vi "Tree_insert tag.vi"(0 "ChannelTree":refnum<vi>, 5 "Active Item:Tag":string, 7 "Left Cell String":string, 9 "Child Text":string[](array[string]), 11 "error in (no error)":errorcluster, 12 "Child Tag":string, 13 "Indent Level (-1 same as ActiveTag)":i32=-1) -> (4 "dup ChannelTree":refnum<vi>, 6 "Active Item:Tag out":string, 8 "Child Position":i32, 15 "error out":errorcluster)   [LabVIEW 2014]
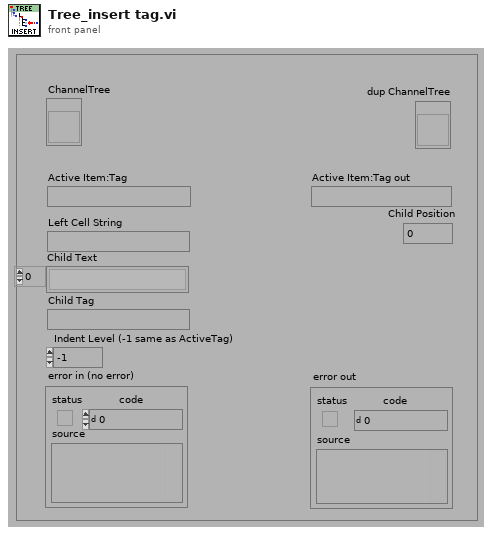
[diagram p1: front panel]
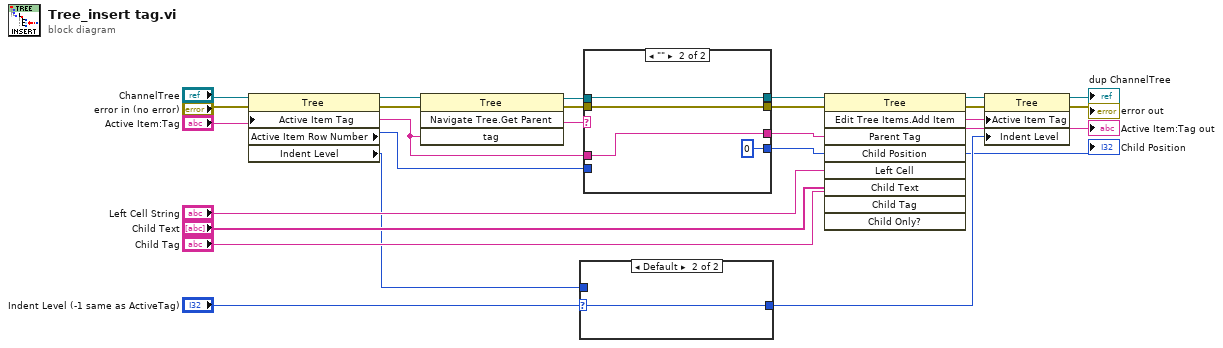
[diagram p0: block diagram]
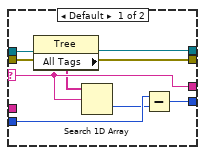
[diagram p2: hidden frame]
diagram:
  n1 = property class="Tree"(reference="ChannelTree", error in="error in (no error)", "Active Item Tag"="Active Item:Tag") -> (reference out=w22:refnum<vi>, error out=w21:errorcluster, "Active Item Row Number"=w8:i32, "Indent Level"=w13:i32)
  n2 = invoke class="Tree" method="Navigate Tree.Get Parent"(reference=w22, error in=w21, "tag"="Active Item:Tag") -> (reference out=w6:refnum<vi>, error out=w5:errorcluster, "Navigate Tree:Get Parent"=w7:string)  [unwired: 1 in, 1 out]
  n3 = case shown="Default" "Indent Level (-1 same as ActiveTag)" {
    selector: "Indent Level (-1 same as ActiveTag)" -> [_ w26]
    tunnel: [w25 w26] -> w18
    tunnel: w13 -> [w25 _]
    frame -1 {
    }
    frame Default {
    }
  }
  n4 = case shown="\"\"" w7 {
    selector: w7 -> [w33 _]
    tunnel: "Active Item:Tag" -> [_ w39]
    tunnel: [w33 w39] -> w12
    tunnel: w8 -> [w35 _]
    tunnel: [w34 0 ("t")] -> w2
    tunnel: w6 -> [w30 w37]
    tunnel: w5 -> [w29 w36]
    tunnel: [w28 w36] -> w4
    tunnel: [w27 w37] -> w3
    frame Default {
      n5 = property class="Tree"(reference=w30, error in=w29) -> (reference out=w27:refnum<vi>, error out=w28:errorcluster, "All Tags"=w31:string[])
      n6 = Search 1D Array(1D array=w31, element=w33) -> (index of element=w32:i32)  [unwired: 1 out]
      n7 = Subtract(x=w35, y=w32) -> (x-y=w34:i32)
    }
    frame "" {
    }
  }
  "Child Position" <- w2
  n8 = invoke class="Tree" method="Edit Tree Items.Add Item"(reference=w3, error in=w4, "Parent Tag"=w12, "Child Position"=w2, "Left Cell"="Left Cell String", "Child Text"="Child Text", "Child Tag"="Child Tag") -> (reference out=w24:refnum<vi>, error out=w23:errorcluster, "Edit Tree Items:Add Item"=w1:string)  [unwired: 2 in, 6 out]
  "Active Item:Tag out" <- w1
  n9 = property class="Tree"(reference=w24, error in=w23, "Active Item Tag"=w1, "Indent Level"=w18) -> (reference out=→"dup ChannelTree":refnum<vi>, error out=→"error out":errorcluster)
